vi "LOC subRemoveTrailingNumbersFromString.vi"(1 "input string":string) -> (0 "output string":string)   [LabVIEW 2020, in "Localization_Tools.lvlib"]
uses:
  Localization_Tools.lvlib
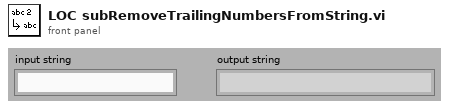
[diagram p1: front panel]
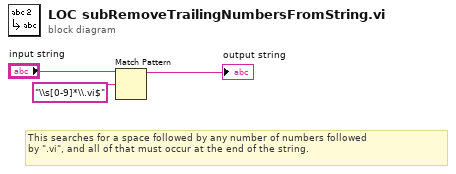
[diagram p0: block diagram]
diagram:
  # "This searches for a space followed by any number of numbers followed\nby \".vi\", and all of that must occur at the end of the string."
  n1 = Match Pattern(string="input string", regular expression="\\s[0-9]*\\.vi$") -> (before substring=→"output string":string)  [unwired: 1 in, 3 out]
